vi "Get Minimal Maximal Size.vi"(7 "Vertical? [F, hor.]":bool, 8 "error in (no error)":errorcluster, 11 "Alternative in":refnum<class "Alternative.lvclass">) -> (0 "error out":errorcluster, 1 "Minimal size":i16, 2 "Maximal size":i16, 3 "IObject out":refnum<class "Alternative.lvclass">)   [LabVIEW 2013, in "Alternative.lvclass"]
doc: "Copyright 2018, Wiebe Walstra, wiebe@carya.nl."
uses:
  Alternative.lvclass
  IObject.lvclass
  IContainer.lvclass
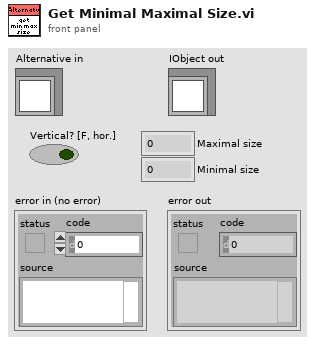
[diagram p1: front panel]
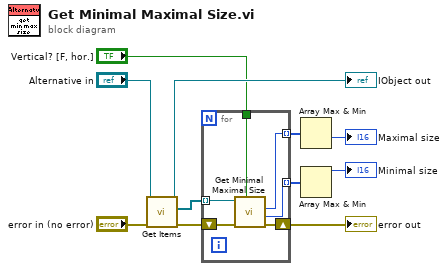
[diagram p0: block diagram]
diagram:
  n1 = call "Get Items.vi"("error in (no error)"="error in (no error)", "IContainer in"="Alternative in") -> ("error out"=w9:errorcluster, "Items"=w6:refnum<class "IObject.lvclass">[], "IContainer out"=→"IObject out":refnum<class "Alternative.lvclass">)  [unwired: 7 in]
  n2 = for {
    tunnel: w6 -> [w15] mode=indexing
    tunnel: "Vertical? [F, hor.]" -> [w14]
    shift-right: [w16] -> w7
    shift-left: w9 -> [w17]
    tunnel: [w13] -> w4 mode=indexing
    tunnel: [w12] -> w2 mode=indexing
    n3 = call-dynamic "Get Minimal Maximal Size.vi"("Vertical? [F, hor.]"=w14, "error in (no error)"=w17, "IObject in"=w15) -> ("error out"=w16:errorcluster, "Minimal size"=w12:i16, "Maximal size"=w13:i16)  [unwired: 5 in, 1 out]
  }
  "error out" <- w7
  n4 = Array Max & Min(array=w4) -> (min value=→"Maximal size":i16)  [unwired: 3 out]
  n5 = Array Max & Min(array=w2) -> (max value=→"Minimal size":i16)  [unwired: 3 out]
